vi "Delete Zero.vi"(8 "error in (no error)":errorcluster, 11 "COBS String in":string) -> (0 "error out":errorcluster, 3 "String out":string)   [LabVIEW 2015, in "LSR Transmission.lvlib"]
uses:
  LSR Transmission.lvlib
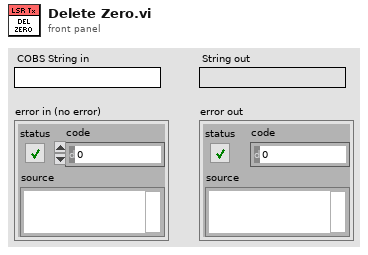
[diagram p1: front panel]
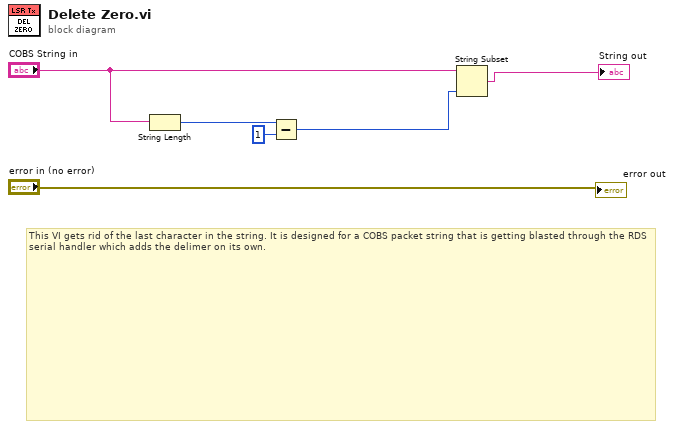
[diagram p0: block diagram]
diagram:
  # "This VI gets rid of the last character in the string. It is designed for a COBS packet string that is getting blasted through the RDS serial handler which adds the delimer on its own."
  n1 = String Length(string="COBS String in") -> (length=w6:i32)
  n2 = Subtract(x=w6, y=1) -> (x-y=w2:i32)
  n3 = String Subset(string="COBS String in", length (rest)=w2) -> (substring=→"String out":string)  [unwired: 1 in]
  "error out" <- "error in (no error)"
